vi "Launch Main.vi"(8 "error in":errorcluster, 10 "Path":path, 11 "Notifier in":refnum<notifier>) -> (0 "error out":errorcluster, 2 "Main Enqueuer":refnum<class "Message Enqueuer.lvclass">, 3 "Notifier out":refnum<notifier>)   [LabVIEW 2023, in "Main.lvlib" / "Main.lvclass"]
uses:
  Project/Main.lvclass
  builds/Engine/Actor Framework.lvlibp/1abvi3w/vi.lib/ActorFramework/Message Enqueuer/Message Enqueuer.lvclass
  C:/Users/Public/Documents/Development/builds/Engine/Engine.lvlibp/Project/Engine.lvclass
  C:/Users/Public/Documents/Development/builds/Engine/Panel Manager.lvlibp/Panel Actor/Panel Actor.lvclass
  builds/Engine/Panel.lvlibp/Window Position/Reference Position/Alignment.ctl
  builds/Engine/Panel.lvlibp/Window Position/Reference Position/Horizontal Alignment.ctl
  builds/Engine/Panel.lvlibp/Window Position/Reference Position/Vertical Alignment.ctl
  builds/Engine/Panel.lvlibp/Window Position/Reference Position/Ref Display/Ref Display.lvclass
  C:/Users/Public/Documents/Development/builds/Engine/Panel.lvlibp/Window Position/Window Position.lvclass
  builds/Engine/Engine.lvlibp/Accessors/Write isRoot.vi
  builds/Engine/Engine.lvlibp/Accessors/Write Directory.vi
  builds/Engine/Panel.lvlibp/Window Position/Reference Position/Ref Display/Ref Display.vi
  builds/Engine/Panel Manager.lvlibp/Panel Actor/Launch Root Panel Window.vi
  builds/Engine/Panel Manager.lvlibp/Panel Actor/Panel Actor.lvclass
  builds/Engine/Panel.lvlibp
  builds/Engine/Panel.lvlibp/Window Position/Reference Position/Reference Position.lvclass
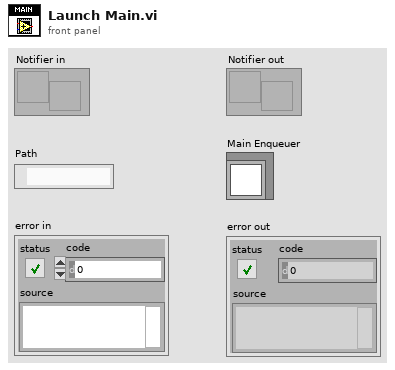
[diagram p1: front panel]
types:
  T1 = typedef "Panel.lvlibp/Reference Position.lvclass/Alignment.ctl" = cluster{"Horizontal":T2, "Vertical":T3}
  T2 = typedef "Panel.lvlibp/Reference Position.lvclass/Horizontal Alignment.ctl" = enum16{"Left", "Center", "Right"}
  T3 = typedef "Panel.lvlibp/Reference Position.lvclass/Vertical Alignment.ctl" = enum16{"Top", "Center", "Bottom"}
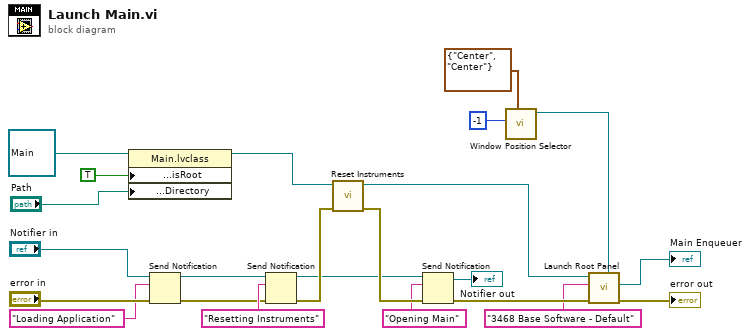
[diagram p0: block diagram]
diagram:
  n1 = property class="Main.lvclass"(reference=refnum<class "Main.lvclass"> refnum ("Base Software.lvlib:Base Software.lvclass"), "Accessors:Application:Information:isRoot"=TRUE ("Engine:App:isRoot"), "Accessors:Application:Information:Directory"="Path") -> (reference out=w15:refnum<class "Main.lvclass">)  [unwired: 1 in, 1 out]
  n2 = Send Notification(notification="Loading Application", notifier="Notifier in", error in (no error)="error in") -> (notifier out=w18:refnum<notifier>, error out=w10:errorcluster)
  n3 = Send Notification(notification="Resetting Instruments", notifier=w18, error in (no error)=w10) -> (notifier out=w9:refnum<notifier>, error out=w21:errorcluster)
  n4 = call "Reset Instruments.vi"("error in"=w21, "Base Software in"=w15) -> ("error out"=w14:errorcluster, "Base Software out"=w7:refnum<class "Main.lvclass">)  [unwired: 8 in]
  n5 = Send Notification(notification="Opening Main", notifier=w9, error in (no error)=w14) -> (notifier out=→"Notifier out":refnum<notifier>, error out=w12:errorcluster)
  n6 = call-poly "Window Position Selector.vi"("Alignment"=T1 {"Horizontal"=enum."Center", "Vertical"=enum."Center"}, "Display (Primary)"=-1) -> ("Ref Display out"=w5:refnum<class "Ref Display.lvclass">)  [unwired: 8 in, 1 out]
  n7 = call-poly "Launch Root Panel.vi"("Window Position (Maximize First Call)"=w5, "Error In"=w12, "Title"="3468 Base Software - Default", "Panel Actor in"=w7) -> ("Error Out"=→"error out":errorcluster, "Actor's Enqueuer"=→"Main Enqueuer":refnum<class "Message Enqueuer.lvclass">)  [unwired: 6 in]
